vi "Display QDFunction Info In QuickBox.vi"(8 "error in (no error)":errorcluster, 11 "NormalQDFunc in":refnum<class "NormalQDFunc.lvclass">) -> (0 "error out":errorcluster, 2 "Content For Display":string, 3 "NormalQDFunc out":refnum<class "NormalQDFunc.lvclass">)   [LabVIEW 2015, in "NormalQDFunc.lvclass"]
uses:
  NormalQDFunc.lvclass
  NormalQDFunc.lvclass/NormalQDFunc.ctl
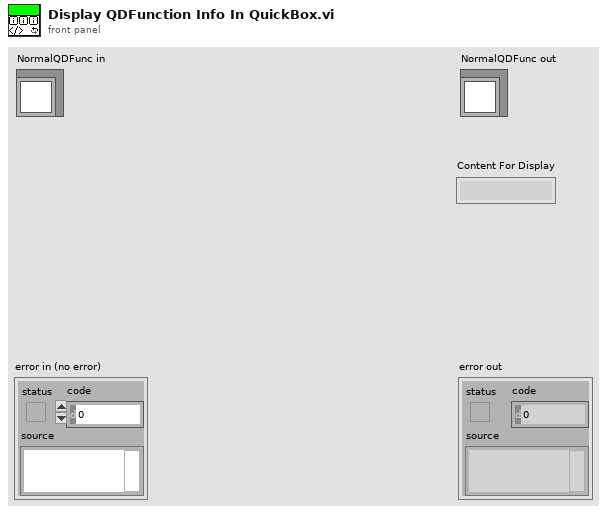
[diagram p1: front panel]
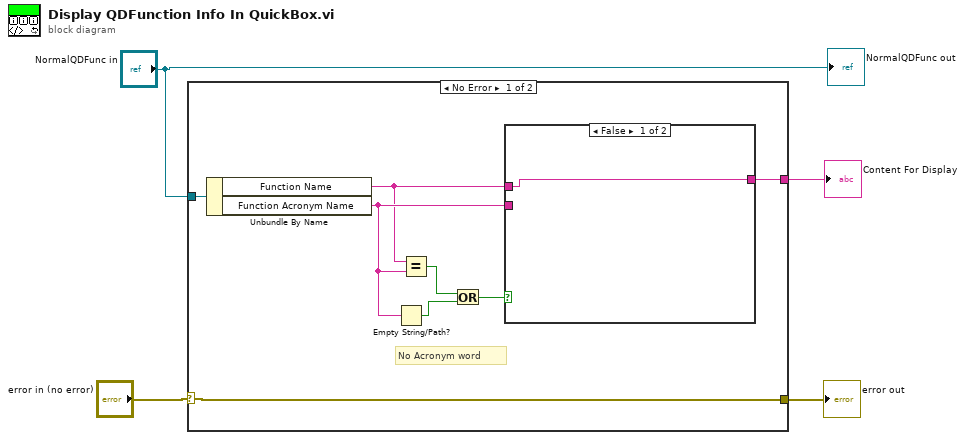
[diagram p0: block diagram]
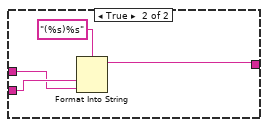
[diagram p2: hidden frame]
diagram:
  n1 = case shown="No Error" "error in (no error)" {
    selector: "error in (no error)" -> [w5 w18]
    tunnel: [w7 _] -> w4
    tunnel: "NormalQDFunc in" -> [w6 _]
    tunnel: [w5 w18] -> w1
    frame No Error {
      # "No Acronym word"
      n2 = Unbundle By Name(w6) -> ("Function Name"=w8:string, "Function Acronym Name"=w9:string)
      n3 = Empty String/Path?(string/path=w9) -> (empty?=w11:bool)
      n4 = Equal?(x=w8, y=w9) -> (x = y?=w12:bool)
      n5 = Or(x=w12, y=w11) -> (x .or. y?=w10:bool)
      n6 = case shown="False" w10 {
        tunnel: w9 -> [_ w16]
        tunnel: w8 -> [w13 w15]
        tunnel: [w13 w14] -> w7
        frame False {
        }
        frame True {
          n7 = Format Into String(format string="(%s)%s", w16, w15) -> (resulting string=w14:string)  [unwired: 2 in, 1 out]
        }
      }
    }
    frame Error {
    }
  }
  "error out" <- w1
  "Content For Display" <- w4
  "NormalQDFunc out" <- "NormalQDFunc in"
